vi "ArmFF_CalculateVelocityOnly.vi"(9 "VelocityRadiansPerSec":dbl, 10 "PositionRadians":dbl, 11 "in ARM_FF":T1 {"kCos" format="%13.5p"; "Ka" format="%13.5p"; "Kv" format="%13.5p"; "Ks" format="%13.5p"}) -> (3 "FeedForward":dbl)   [LabVIEW 2019, in "Trajectory_Library.lvlib"]
doc: "Calculates the feedforward from the gains and velocity setpoint (acceleration is assumed to be zero).\n \nInputs: \n - ArmFF -- The ArmFF data cluster\n - positionRadians -- The position (angle) setpoint.\n - velocity -- The velocity setpoint.\n\nOutputs:\n - feedForward -- The computed feedforward."
uses:
  Trajectory_Library.lvlib
  TypeDef/ARM_FF.ctl
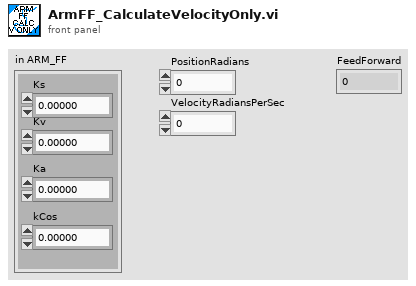
[diagram p1: front panel]
types:
  T1 = typedef "Trajectory_Library.lvlib/ARM_FF.ctl" = cluster{"Ks":dbl, "Kv":dbl, "Ka":dbl, "kCos":dbl}
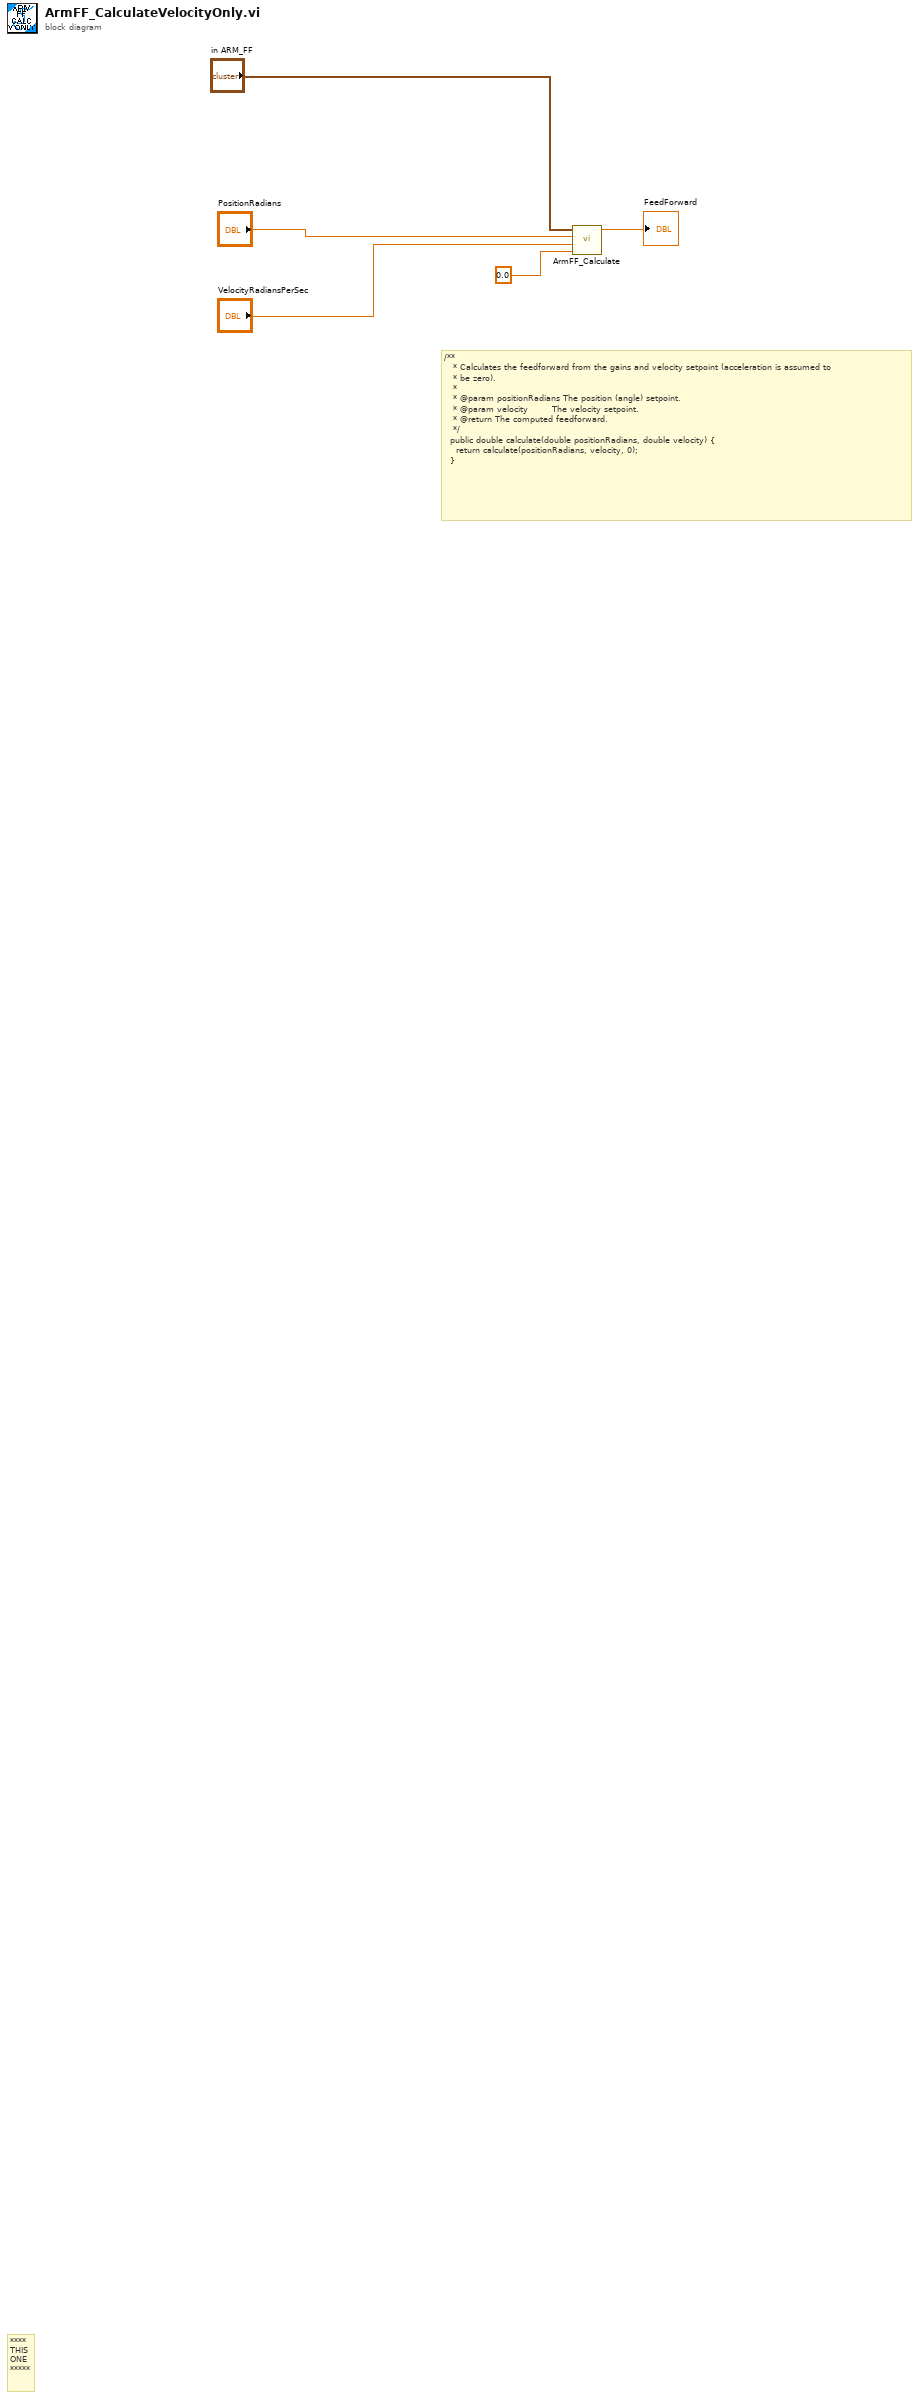
[diagram p0: block diagram]
diagram:
  # "/**\n   * Calculates the feedforward from the gains and velocity setpoint (acceleration is assumed to\n   * be zero).\n   *\n   * @param positionRadians The position (angle) setpoint.\n   * @param velocity        The velocity setpoint.\n   * @return The computed feedforward.\n   */\n  public double calculate(double positionRadians, double velocity) {\n    return calculate(positionRadians, velocity, 0);\n  }"
  # "****\nTHIS\nONE\n*****"
  n1 = call "ArmFF_Calculate.vi"("AccelRadPerSecSquared"=0.0, "VelocityRadiansPerSec"="VelocityRadiansPerSec", "PositionRadians"="PositionRadians", "in ARM_FF"="in ARM_FF") -> ("FeedForward"=→"FeedForward":dbl)  [unwired: 7 in]
